vi "MouseUp Response.vi"(4 "PlatMods":T1, 6 "Mods":cluster{"Double Click":bool, "Menu Key":bool}, 8 "error in (no error)":errorcluster, 9 "Button":u16, 10 "Coords":T2, 11 "Editor Handler in":refnum<class "Image Editor Handler.lvclass">) -> (0 "error out":errorcluster, 3 "Editor Handler out":refnum<class "Image Editor Handler.lvclass">)   [LabVIEW 2015, in "LV Image Editor Framework.lvlib" / "Image Editor Handler.lvclass"]
uses:
  Image Editor Handler.lvclass
  <vilib>/Utility/miscctls.llb/LVPoint32TypeDef.ctl
  Image Editor Handler.lvclass/Image Editor Handler.ctl
  Forms/Shape/Shape.lvclass
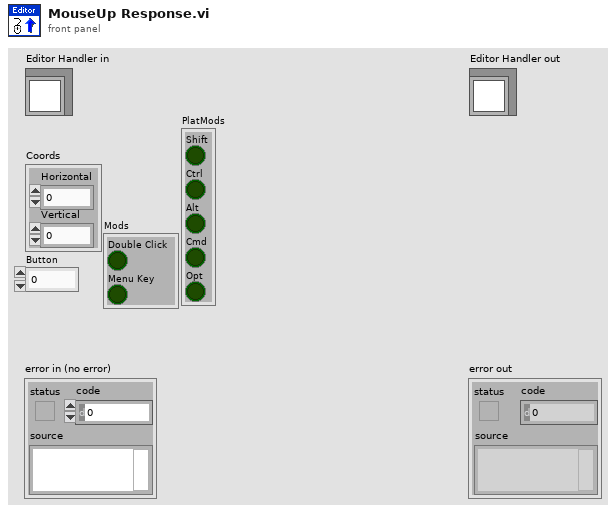
[diagram p1: front panel]
types:
  T1 = cluster{"Shift":bool, "Ctrl":bool, "Alt":bool, "Cmd":bool, "Opt":bool}
  T2 = typedef "LVPoint32TypeDef.ctl" = cluster{"Horizontal":i32, "Vertical":i32}
  T3 = typedef "LVPositionTypeDef.ctl" = cluster{"Left":i32, "Top":i32}
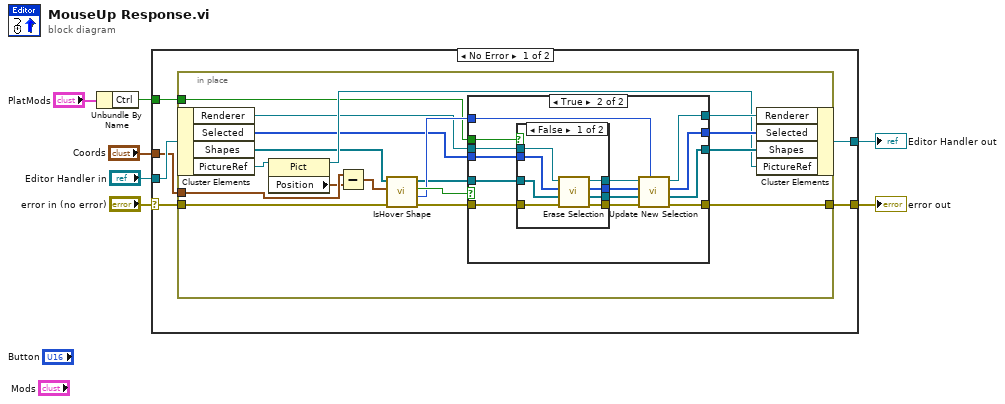
[diagram p0: block diagram]
diagram:
  n1 = Unbundle By Name("PlatMods") -> ("Ctrl"=w2:bool)
  n2 = case shown="No Error" "error in (no error)" {
    selector: "error in (no error)" -> [w9 w63]
    tunnel: [w8 w63] -> w6
    tunnel: [w11 w62] -> w4
    tunnel: "Editor Handler in" -> [w13 w62]
    tunnel: w2 -> [w10 _]
    tunnel: "Coords" -> [w12 _]
    frame No Error {
      n3 = in-place {
        in-place-border: w12 -> [w30]
        in-place-border: w10 -> [w17]
        in-place-border: w9 -> [w16]
        in-place-border: [w14] -> w8
        n4 = in-place-cluster #1(w13) -> ("Renderer"=w21:refnum<class "Image.lvclass">, "Selected"=w20:i16[], "Shapes"=w19:refnum<data-value>[], "PictureRef"=w31:refnum<vi>)
        n5 = property class="Pict"(reference=w31) -> (reference out=w22:refnum<vi>, "Position"=w29:T3)  [unwired: 1 in, 1 out]
        n6 = Subtract(x=w30, y=w29) -> (x-y=w28:T2)
        n7 = call "IsHover Shape.vi"("error in (no error)"=w16, "Coords"=w28, "Shape in"=w19) -> ("error out"=w15:errorcluster, "Node ID"=w25:i32, "Found?"=w27:bool, "Shape out"=w18:refnum<data-value>[])  [unwired: 3 in, 2 out]
        n8 = case shown="True" w27 {
          tunnel: w21 -> [w35 w45]
          tunnel: [w35 w49] -> w26
          tunnel: w20 -> [w34 w41]
          tunnel: w25 -> [_ w48]
          tunnel: [w33 w47] -> w24
          tunnel: [w34 w46] -> w23
          tunnel: w18 -> [w33 w40]
          tunnel: w17 -> [_ w39]
          tunnel: w15 -> [w32 w38]
          tunnel: [w32 w36] -> w14
          frame False {
          }
          frame True {
            n9 = case shown="False" w39 {
              tunnel: w45 -> [w57 w61]
              tunnel: [w56 w60] -> w44
              tunnel: [w55 w59] -> w43
              tunnel: [w54 w61] -> w42
              tunnel: w41 -> [w53 w60]
              tunnel: w40 -> [w52 w59]
              tunnel: w38 -> [w51 w58]
              tunnel: [w50 w58] -> w37
              frame False {
                n10 = call "Erase Selection.vi"("error in (no error)"=w51, "Shape in"=w52, "Selected in"=w53, "Image in"=w57) -> ("error out"=w50:errorcluster, "Shape out"=w55:refnum<data-value>[], "Selected out"=w56:i16[], "Image out"=w54:refnum<class "Image.lvclass">)  [unwired: 4 in]
              }
              frame True {
              }
            }
            n11 = call "Update New Selection.vi"("Node ID"=w48, "error in (no error)"=w37, "Shape in"=w43, "Selected in"=w44, "Image in"=w42) -> ("error out"=w36:errorcluster, "Shape out 2"=w47:refnum<data-value>[], "Selected out 2"=w46:i16[], "Image out"=w49:refnum<class "Image.lvclass">)  [unwired: 3 in]
          }
        }
        n12 = in-place-cluster #1("Renderer"=w26, "Selected"=w23, "Shapes"=w24, "PictureRef"=w22) -> (w11:refnum<class "Image Editor Handler.lvclass">)
      }
    }
    frame Error {
    }
  }
  "error out" <- w6
  "Editor Handler out" <- w4
